vi "Initialize with copy transmission.vi"(8 "error in (no error)":errorcluster, 9 "unit ID":u8=1, 10 "MB copy":refnum<class "Master CR.lvclass">, 11 "MB in":refnum<class "Master CR.lvclass">) -> (0 "error out":errorcluster, 3 "MB out":refnum<class "Master CR.lvclass">)   [LabVIEW 2021, in "Master CR.lvclass"]
uses:
  Master CR.lvclass
  Master CR.lvclass/Master CR.ctl
  Modbus_v121c/Data Model/Device Data Model.lvclass
  Modbus_v121c/Network Protocol/Network Master/Network Master.lvclass
  D:/my_projects/projects/Algorithms/Labview/21/Modbus_v121c/Network Protocol/Network Protocol.lvclass
  D:/my_projects/projects/Algorithms/Labview/21/Modbus_v121c/Network Protocol/Network Master/Network Master.lvclass
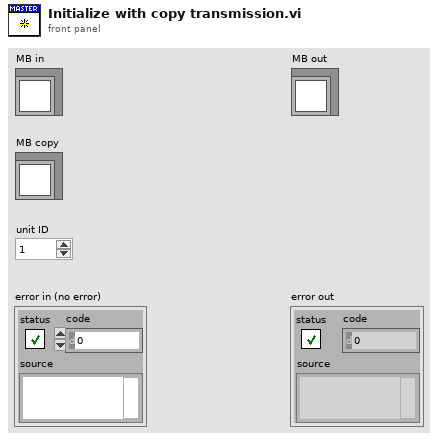
[diagram p1: front panel]
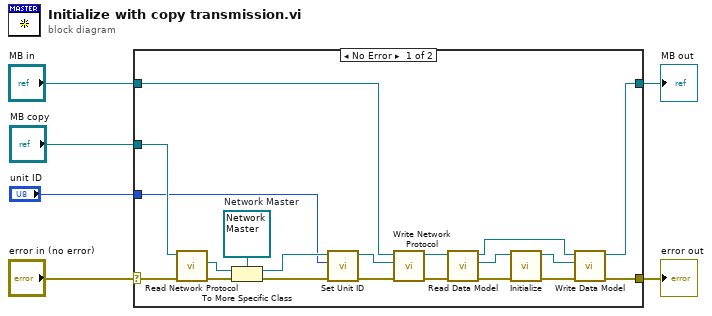
[diagram p0: block diagram]
diagram:
  n1 = case shown="No Error" "error in (no error)" {
    selector: "error in (no error)" -> [w19 w27]
    tunnel: [w20 w27] -> w5
    tunnel: [w21 w28] -> w3
    tunnel: "MB in" -> [w9 w28]
    tunnel: "MB copy" -> [w18 _]
    tunnel: "unit ID" -> [w12 _]
    frame No Error {
      w16 = refnum<class "Network Master.lvclass"> refnum  # Network Master
      n2 = call "Read Network Protocol.vi"("error in (no error)"=w19, "Master CR in"=w18) -> ("error out"=w17:errorcluster, "Network Protocol"=w15:refnum<class "Network Protocol.lvclass">)  [unwired: 7 in, 1 out]
      n3 = To More Specific Class(target class=w16, reference=w15, error in=w17) -> (specific class reference=w14:refnum<class "Network Master.lvclass">, error out=w13:errorcluster)
      n4 = call "Set Unit ID.vi"("error in (no error)"=w13, "Unit ID"=w12, "Modbus master in"=w14) -> ("error out"=w10:errorcluster, "Modbus master out"=w11:refnum<class "Network Master.lvclass">)  [unwired: 7 in]
      n5 = call "Write Network Protocol.vi"("error in (no error)"=w10, "Network Protocol"=w11, "Master CR in"=w9) -> ("error out"=w7:errorcluster, "Master CR out"=w8:refnum<class "Master CR.lvclass">)  [unwired: 7 in]
      n6 = call "Read Data Model.vi"("error in (no error)"=w7, "Master CR in"=w8) -> ("error out"=w25:errorcluster, "Data Model"=w26:refnum<class "Device Data Model.lvclass">, "Master CR out"=w22:refnum<class "Master CR.lvclass">)  [unwired: 7 in]
      n7 = call-dynamic "Initialize.vi"("error in"=w25, "device data model in"=w26) -> ("error out"=w24:errorcluster, "device data model out"=w23:refnum<class "Device Data Model.lvclass">)  [unwired: 8 in]
      n8 = call "Write Data Model.vi"("error in (no error)"=w24, "Data Model"=w23, "Master CR in"=w22) -> ("error out"=w20:errorcluster, "Master CR out"=w21:refnum<class "Master CR.lvclass">)  [unwired: 7 in]
    }
    frame Error {
    }
  }
  "error out" <- w5
  "MB out" <- w3
